vi "Roll dice.vi"() -> ()   [LabVIEW 2018]
panel:
  in  "정지":bool
  in  "출력":bool
  out "슬라이드":dbl(slide) scale=1.0..6.0
  out "미터":dbl(knob) scale=1.0..6.0
  out "주사위 랜덤추출기":dbl
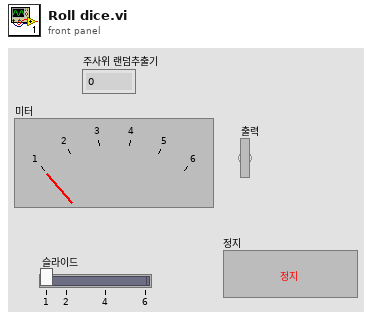
[diagram p1: front panel]
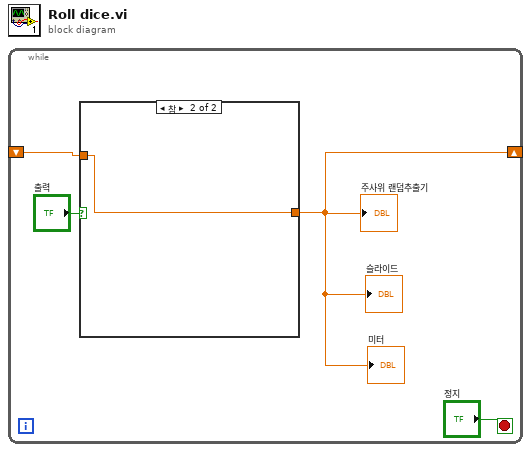
[diagram p0: block diagram]
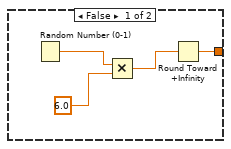
[diagram p2: hidden frame]
diagram:
  n1 = while {
    shift-right: [w2] -> _
    shift-left: _ -> [w1]
    stop <- "정지" stop-if-true
    n2 = case shown="참" "출력" {
      tunnel: [w5 w9] -> w2
      tunnel: w1 -> [_ w9]
      frame False {
        n3 = Random Number (0-1)() -> (number: 0 to 1=w7:dbl)
        n4 = Multiply(x=w7, y=6.0) -> (x*y=w8:dbl)
        n5 = Round Toward +Infinity(x=w8) -> (ceil(x): smallest int >= x=w5:dbl)
      }
      frame True {
      }
    }
    "주사위 랜덤추출기" <- w2
    "미터" <- w2
    "슬라이드" <- w2
  }
